vi "trash test ftp issues.vi"() -> ()   [LabVIEW 2010]
uses:
  FTP Credintials.ctl
  <vilib>/addons/internet/NI_InternetTK_FTP_VIs.lvlib
panel:
  out "Array 3":bool[](array[boolean])
  out "Array 2":string[](array[string])
  out "Array":cluster{"name":string, "Equal File size":bool}[](array[cluster])
  in  "Directory Path":path
  in  "File Pattern (*.CSV .ddf)":string
  in  "FTP Creds":T1 {"FTP Timeout (S)" min=0 max=10 step=1}
  in  "active (T)":bool=TRUE
  out "error out":errorcluster
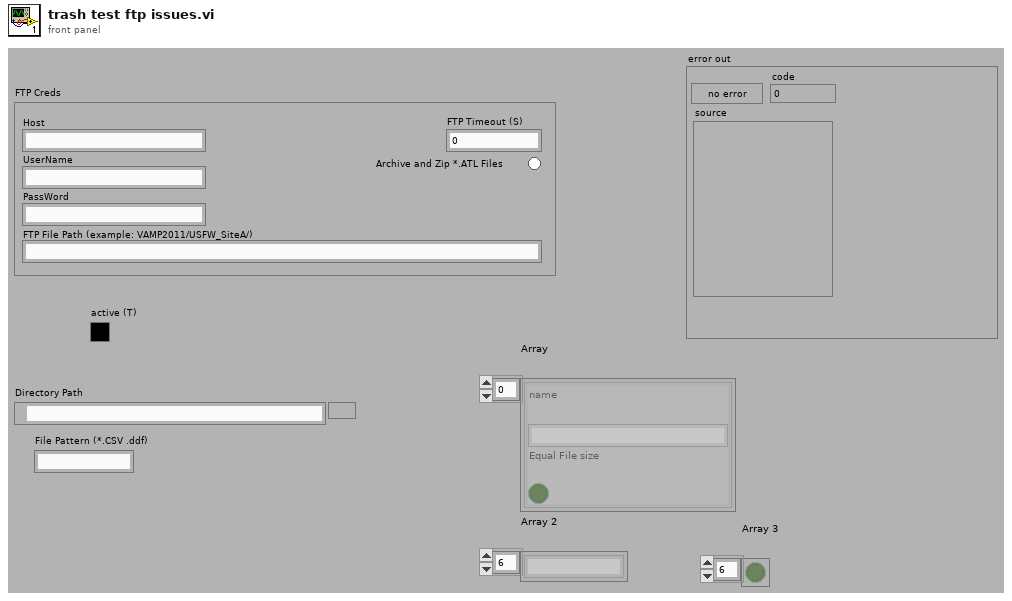
[diagram p1: front panel]
types:
  T1 = typedef "FTP Credintials.ctl" = cluster{"Host":string, "UserName":string, "PassWord":string, "FTP File Path":string, "FTP Timeout (S)":i32, "Use ATL":bool}
  T2 = typedef "FTP Session.ctl" = refnum<k1>
  T3 = typedef "FTP File Info.ctl" = cluster{"type":enum16{"unknown", "file", "dir", "link"}, "permissions":string, "owner":string, "group":string, "size":i32, "date":string, "name":string, "link name":string}
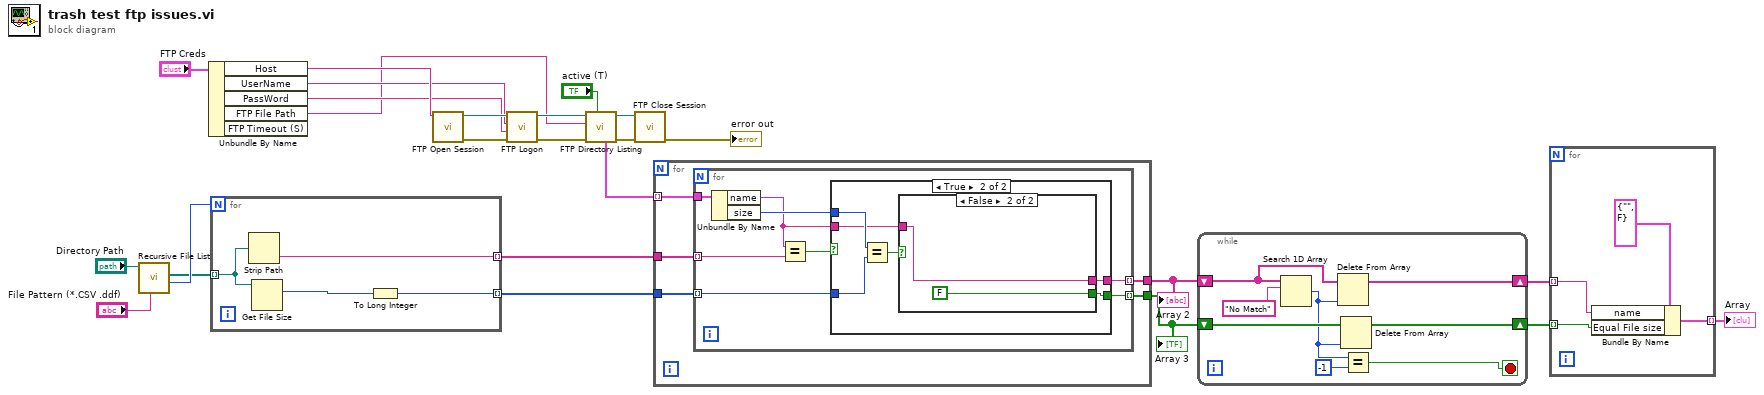
[diagram p0: block diagram]
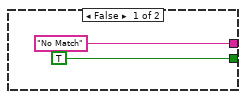
[diagram p2: hidden frame]
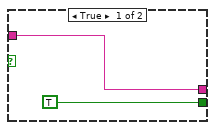
[diagram p3: hidden frame]
diagram:
  n1 = call <vilib>:"Recursive File List.vi"("pattern"="File Pattern (*.CSV .ddf)", "Folder Path"="Directory Path") -> ("Number of Files"=w12:i32, "All Files in Dir"=w11:path[])  [unwired: 5 in, 3 out]
  n2 = Unbundle By Name("FTP Creds") -> ("Host"=w16:string, "UserName"=w15:string, "PassWord"=w14:string, "FTP File Path"=w13:string)  [unwired: 1 out]
  n3 = for {
    N: w12 -> [_]
    tunnel: w11 -> [w29] mode=indexing
    tunnel: [w28] -> w7 mode=indexing
    tunnel: [w26] -> w6 mode=indexing
    n4 = Strip Path(path=w29) -> (name=w28:string)  [unwired: 1 out]
    n5 = Get File Size(file=w29) -> (size (in bytes)=w27:i64)  [unwired: 1 in, 2 out]
    n6 = To Long Integer(number=w27) -> (32bit integer=w26:i32)
  }
  n7 = call <vilib>:"FTP Open Session.vi"("address"=w16) -> ("error out"=w24:errorcluster, "ftp session"=w25:T2)  [unwired: 7 in, 2 out]
  n8 = call <vilib>:"FTP Logon.vi"("error in (no error)"=w24, "password"=w14, "user"=w15, "ftp session"=w25) -> ("error out"=w21:errorcluster, "ftp session out"=w22:T2)  [unwired: 4 in, 2 out]
  n9 = call <vilib>:"FTP Directory Listing.vi"("active (T)"="active (T)", "error in (no error)"=w21, "directory path"=w13, "ftp session"=w22) -> ("error out"=w18:errorcluster, "ftp session out"=w19:T2, "dir list"=w8:T3[])  [unwired: 3 in, 2 out]
  n10 = call <vilib>:"FTP Close Session.vi"("error in (no error)"=w18, "ftp session"=w19) -> ("error out"=→"error out":errorcluster)  [unwired: 6 in, 3 out]
  n11 = for {
    tunnel: w8 -> [w34] mode=indexing
    tunnel: w7 -> [w33]
    tunnel: w6 -> [w32]
    tunnel: [w31] -> w5
    tunnel: [w30] -> w4
    n12 = for {
      tunnel: w34 -> [w42]
      tunnel: w33 -> [w40] mode=indexing
      tunnel: w32 -> [w38] mode=indexing
      tunnel: [w36] -> w31 mode=indexing
      tunnel: [w35] -> w30 mode=indexing
      n13 = Unbundle By Name(w42) -> ("name"=w37:string, "size"=w39:i32)
      n14 = Equal?(x=w37, y=w40) -> (x = y?=w41:bool)
      n15 = case shown="True" w41 {
        tunnel: w39 -> [_ w49]
        tunnel: w38 -> [_ w48]
        tunnel: w37 -> [_ w47]
        tunnel: ["No Match" ("name") w45] -> w36
        tunnel: [TRUE w46] -> w35
        frame False {
        }
        frame True {
          n16 = Equal?(x=w49, y=w48) -> (x = y?=w50:bool)
          n17 = case shown="False" w50 {
            tunnel: w47 -> [w51 w53]
            tunnel: [TRUE FALSE] -> w46
            tunnel: [w51 w53] -> w45
            frame True {
            }
            frame False {
            }
          }
        }
      }
    }
  }
  "Array 2" <- w5
  "Array 3" <- w4
  n18 = while {
    shift-right: [w56] -> w3
    shift-left: w5 -> [w61]
    shift-right: [w55] -> w2
    shift-left: w4 -> [w60]
    stop <- w57 stop-if-true
    n19 = Search 1D Array(1D array=w61, element="No Match" ("name")) -> (index of element=w59:i32)  [unwired: 1 in]
    n20 = Delete From Array(array=w61, index=w59) -> (array with subset deleted=w56:string[])  [unwired: 1 in, 1 out]
    n21 = Delete From Array(array=w60, index=w59) -> (array with subset deleted=w55:bool[])  [unwired: 1 in, 1 out]
    n22 = Equal?(x=w59, y=-1) -> (x = y?=w57:bool)
  }
  n23 = for {
    tunnel: w3 -> [w65] mode=indexing
    tunnel: w2 -> [w64] mode=indexing
    tunnel: [w63] -> w1 mode=indexing
    n24 = Bundle By Name(cluster=cluster{"name":string, "Equal File size":bool} {"name"="", "Equal File size"=FALSE} ("input cluster"), "name"=w65, "Equal File size"=w64) -> (w63:cluster{"name":string, "Equal File size":bool})
  }
  "Array" <- w1
